vi "Priority.vi"(8 "error in (no error)":errorcluster, 11 "NoControllerException in":refnum<class "NoControllerException.lvclass">) -> (0 "error out":errorcluster, 2 "Priority":u16, 3 "NoControllerException out":refnum<class "NoControllerException.lvclass">)   [LabVIEW 2020, in "HTTP Server.lvlib" / "NoControllerException.lvclass"]
uses:
  NoControllerException.lvclass
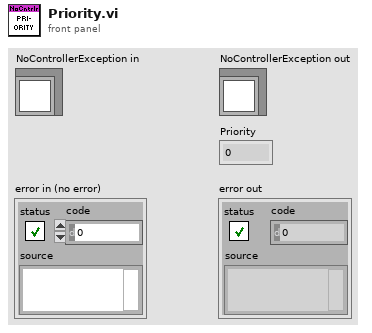
[diagram p1: front panel]
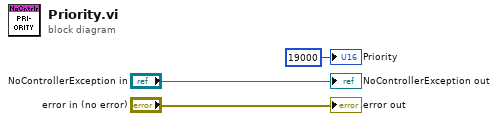
[diagram p0: block diagram]
diagram:
  "error out" <- "error in (no error)"
  "NoControllerException out" <- "NoControllerException in"
  "Priority" <- u16 19000 ("Priority")
